vi "Test Perform Action.vi"(11 "Test Case In":refnum<class "NI9476 Fixed Freq PWM CFG.lvclass">) -> (0 "error out":errorcluster, 3 "Test Case Out":refnum<class "NI9476 Fixed Freq PWM CFG.lvclass">)   [LabVIEW 2024, in "NI9476 Fixed Freq PWM CFG.lvclass"]
uses:
  NI9476 Fixed Freq PWM CFG.lvclass
  NI9476 Fixed Freq PWM CFG.lvclass/NI9476 Fixed Freq PWM CFG.ctl
  <vilib>/Astemes/LUnit/Test Case.lvclass
  0b62ffe9-8e84-4b56-bf2a-6d3c5537c85a.vi
  HAL/Configurations/CFG Base/CFG Base.lvclass
  HAL/Devices/DAQmx/DIO/DI DAQmx Cont CFG/DI DAQmx Cont CFG.lvclass
  D:/git/HAL/HAL/Devices/DAQmx/DAQmx Base CFG/DAQmx Base CFG.lvclass
  D:/git/HAL/HAL/Configurations/CFG Base/CFG Base.lvclass
  D:/git/HAL/HAL/Devices/DAQmx/DIO/DI DAQmx Cont CFG/DI DAQmx Cont CFG.lvclass
  C:/Program Files/National Instruments/LabVIEW 2024/vi.lib/Astemes/LUnit/Test Case.lvclass
  C:/Program Files/National Instruments/LabVIEW 2024/vi.lib/Astemes/LUnit/LUnit Runnable.lvclass
  D:/git/HAL/Tests/NI9476 Fixed Freq PWM CFG/NI9476 Fixed Freq PWM CFG.lvclass
panel:
  out "error out 2":errorcluster
  out "Array":variant[](array[variant])
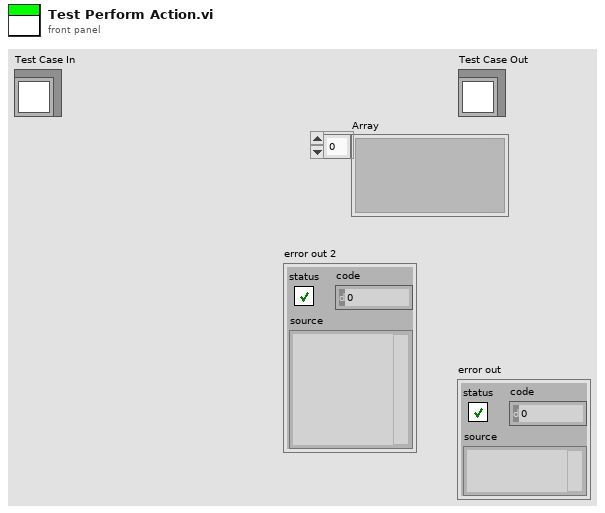
[diagram p1: front panel]
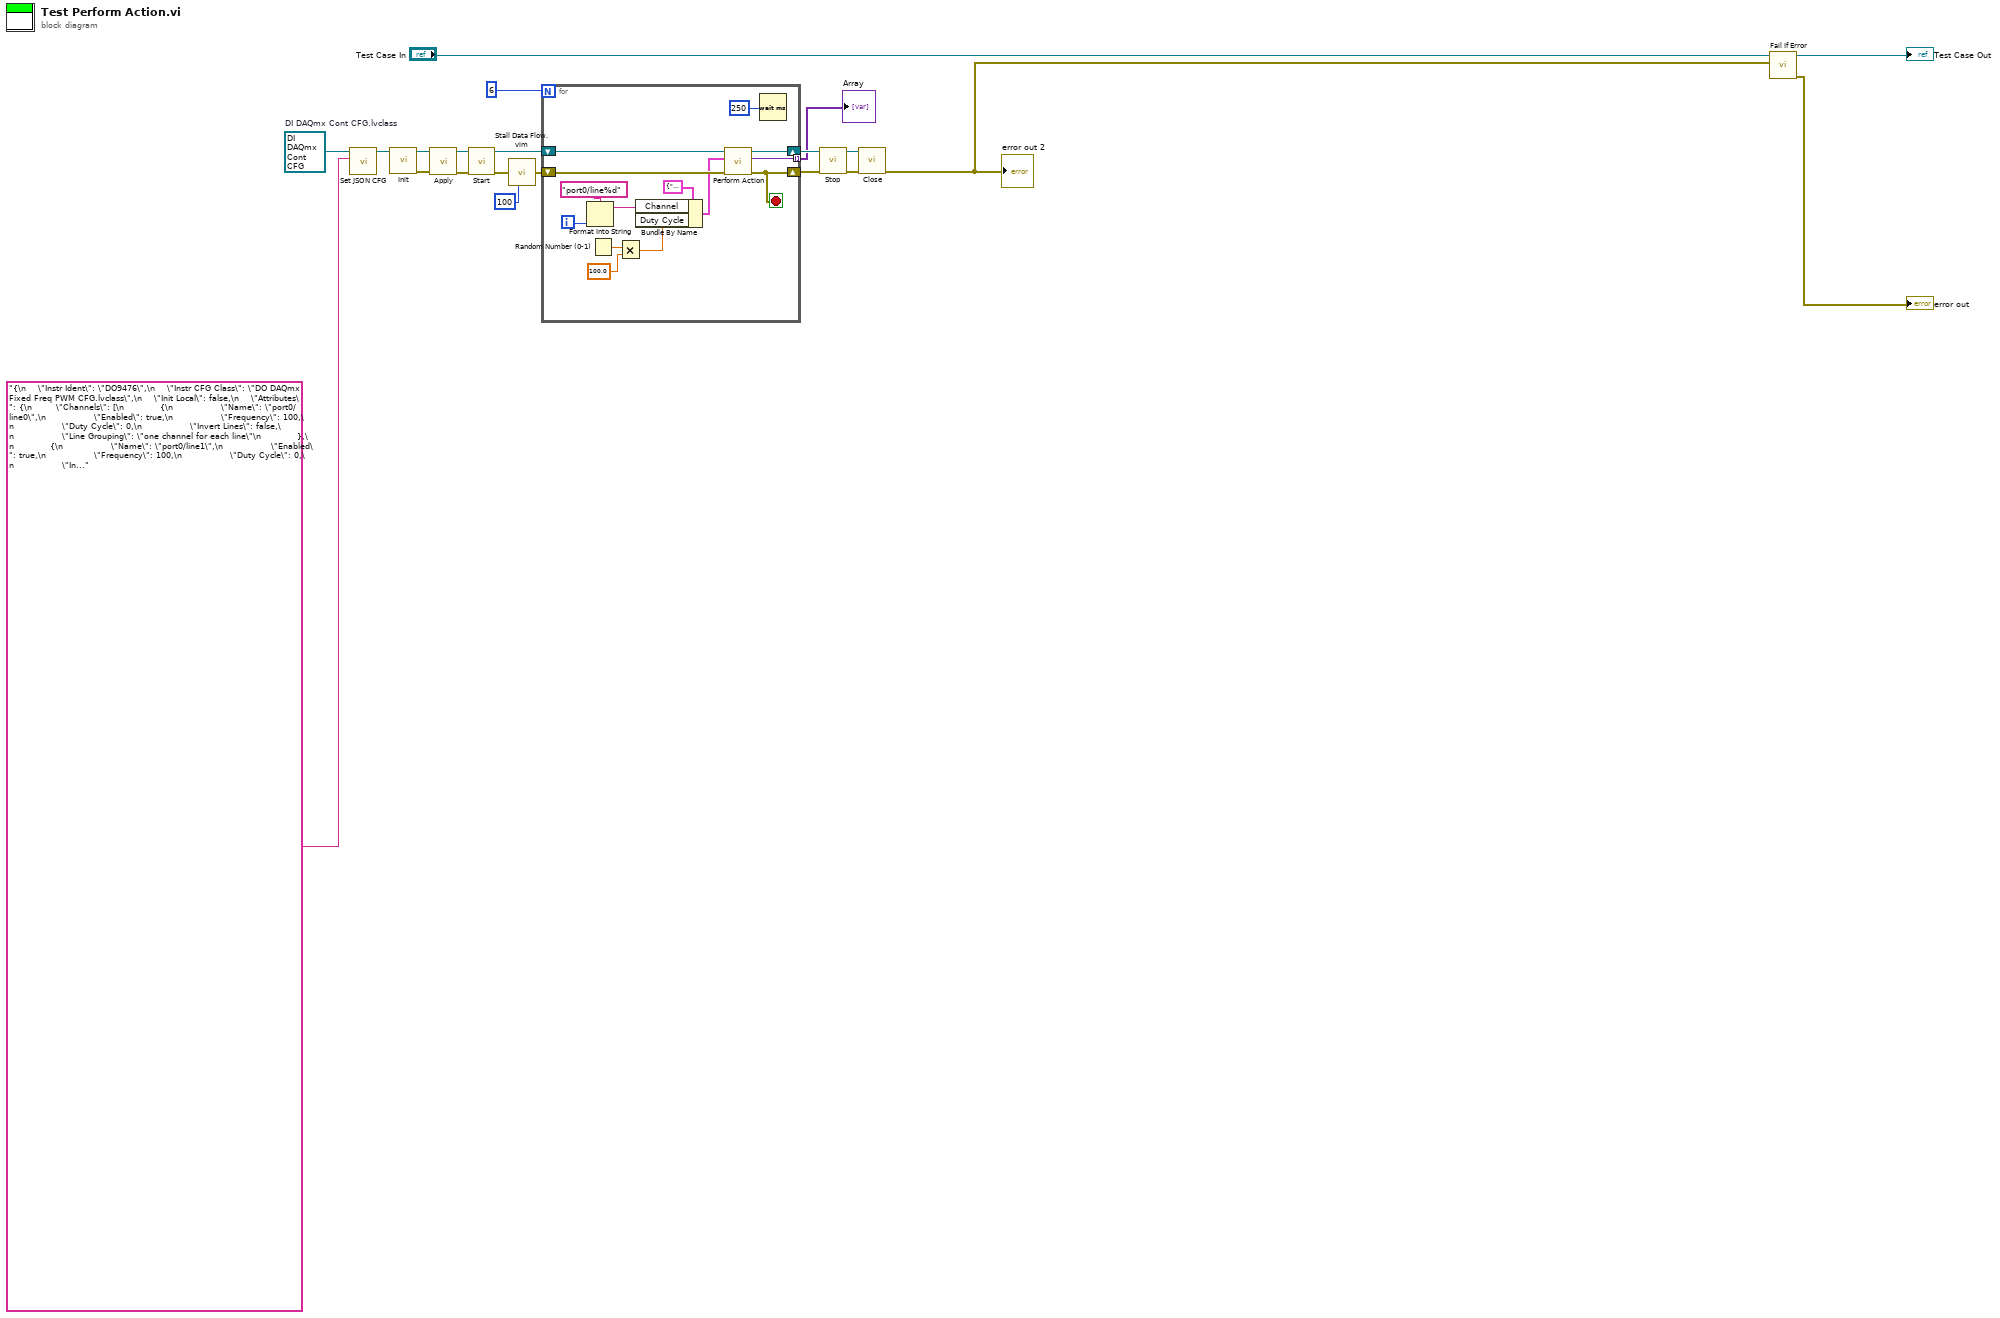
[diagram p0: block diagram]
diagram:
  w1 = refnum<class "DI DAQmx Cont CFG.lvclass"> refnum  # DI DAQmx Cont CFG.lvclass
  n1 = call "Set JSON CFG.vi"("<JSON>CFG"="{\n    \"Instr Ident\": \"DO9476\",\n    \"Instr CFG Class\": \"DO DAQmx Fixed Freq PWM CFG.lvclass\",\n    \"Init Local\": false,\n    \"Attributes\": {\n        \"Channels\": [\n            {\n                \"Name\": \"port0/line0\",\n                \"Enabled\": true,\n                \"Frequency\": 100,\n                \"Duty Cycle\": 0,\n                \"Invert Lines\": false,\n                \"Line Grouping\": \"one channel for each line\"\n            },\n            {\n                \"Name\": \"port0/line1\",\n                \"Enabled\": true,\n                \"Frequency\": 100,\n                \"Duty Cycle\": 0,\n                \"Invert Lines\": false,\n                \"Line Grouping\": \"one channel for each line\"\n            },\n            {\n                \"Name\": \"port0/line2\",\n                \"Enabled\": true,\n                \"Frequency\": 100,\n                \"Duty Cycle\": 0,\n                \"Invert Lines\": false,\n                \"Line Grouping\": \"one channel for each line\"\n            },\n            {\n                \"Name\": \"port0/line3\",\n                \"Enabled\": true,\n                \"Frequency\": 100\n                \"Duty Cycle\": 0,\n                \"Invert Lines\": false,\n                \"Line Grouping\": \"one channel for each line\"\n            },\n            {\n                \"Name\": \"port0/line4\",\n                \"Enabled\": true,\n                \"Frequency\": 100,\n                \"Duty Cycle\": 0,\n                \"Invert Lines\": false,\n                \"Line Grouping\": \"one channel for each line\"\n            },\n            {\n                \"Name\": \"port0/line5\",\n                \"Enabled\": true,\n                \"Frequency\": 100,\n                \"Duty Cycle\": 0,\n                \"Invert Lines\": false,\n                \"Line Grouping\": \"one channel for each line\"\n            }\n        ],\n        \"Timing\": {\n            \"Type\": \"Sample Clock\",\n            \"Samples per Channel\": 400,\n            \"Sample Mode\": \"Continuous Samples\",\n            \"Sample Rate\": 2000,\n            \"Sample Clock Source\": \"OnboardClock\",\n            \"Active Edge\": \"Rising\"\n        },\n        \"Trigger\": {\n            \"Trigger Type\": \"No Trigger\"\n        },\n        \"Generation\": {\n            \"Regen Mode\": \"Allow Regeneration\"\n        }\n    }\n}" ("<JSON> CFG"), "CFG Base in"=w1) -> ("CFG Base out"=w8:refnum<class "DI DAQmx Cont CFG.lvclass">)  [unwired: 9 in]
  n2 = call-dynamic "Init.vi"("DAQmx Base CFG in"=w8) -> ("error out"=w18:errorcluster, "DAQmx Base CFG out"=w7:refnum<class "DI DAQmx Cont CFG.lvclass">)  [unwired: 9 in]
  n3 = call-dynamic "Apply.vi"("error in"=w18, "DAQmx Base CFG in"=w7) -> ("error out"=w16:errorcluster, "DAQmx Base CFG out"=w15:refnum<class "DI DAQmx Cont CFG.lvclass">)  [unwired: 8 in]
  n4 = call-dynamic "Start.vi"("error in"=w16, "DAQmx Base CFG in"=w15) -> ("error out"=w13:errorcluster, "DAQmx Base CFG out"=w14:refnum<class "DI DAQmx Cont CFG.lvclass">)  [unwired: 8 in]
  n5 = call "Stall Data Flow.vim"("value in"=w13, "milliseconds to wait"=u32 100) -> ("value out"=w3:errorcluster)  [unwired: 1 out]
  n6 = for {
    N: 6 -> [_]
    shift-right: [w31] -> w11
    shift-left: w3 -> [w34]
    shift-right: [w33] -> w12
    shift-left: w14 -> [w35]
    tunnel: [w22] -> w5 mode=indexing
    i -> [w27]
    stop <- w31 stop-if-true
    n7 = Format Into String(format string="port0/line%d", w27) -> (resulting string=w29:string)  [unwired: 2 in, 1 out]
    n8 = Random Number (0-1)() -> (number: 0 to 1=w26:dbl)
    n9 = Multiply(x=w26, y=100.0) -> (x*y=w24:dbl)
    n10 = Bundle By Name(cluster=cluster{"Channel":string, "Duty Cycle":dbl} {"Channel"="", "Duty Cycle"=0.0}, "Channel"=w29, "Duty Cycle"=w24) -> (w23:cluster{"Channel":string, "Duty Cycle":dbl})
    n11 = call-dynamic "Perform Action.vi"("error in"=w34, "Input"=w23, "CFG Base in"=w35) -> ("error out"=w31:errorcluster, "Output"=w22:variant, "CFG Base out"=w33:refnum<class "DI DAQmx Cont CFG.lvclass">)  [unwired: 6 in]
    n12 = Wait (ms)(milliseconds to wait=u32 250) -> ()  [unwired: 1 out]
  }
  "Array" <- w5
  n13 = call-dynamic "Stop.vi"("error in"=w11, "DAQmx Base CFG in"=w12) -> ("error out"=w10:errorcluster, "DAQmx Base CFG out"=w9:refnum<class "DI DAQmx Cont CFG.lvclass">)  [unwired: 8 in]
  n14 = call-dynamic "Close.vi"("error in"=w10, "DAQmx Base CFG in"=w9) -> ("error out"=w4:errorcluster)  [unwired: 8 in, 1 out]
  "error out 2" <- w4
  n15 = call <vilib>:"Fail If Error.vi"("Assert error"=w4, "LUnit Test Case In"="Test Case In") -> ("error out"=→"error out":errorcluster, "LUnit Test Case Out"=→"Test Case Out":refnum<class "NI9476 Fixed Freq PWM CFG.lvclass">)  [unwired: 8 in]
